vi "Read State.vi"(8 "error in (no error)":errorcluster, 11 "Monitor in":refnum<class "Monitor.lvclass">) -> (0 "error out":errorcluster, 2 "State":bool, 3 "Monitor out":refnum<class "Monitor.lvclass">)   [LabVIEW 2016, in "Monitor.lvclass"]
uses:
  Monitor.lvclass
  Monitor.lvclass/Monitor.ctl
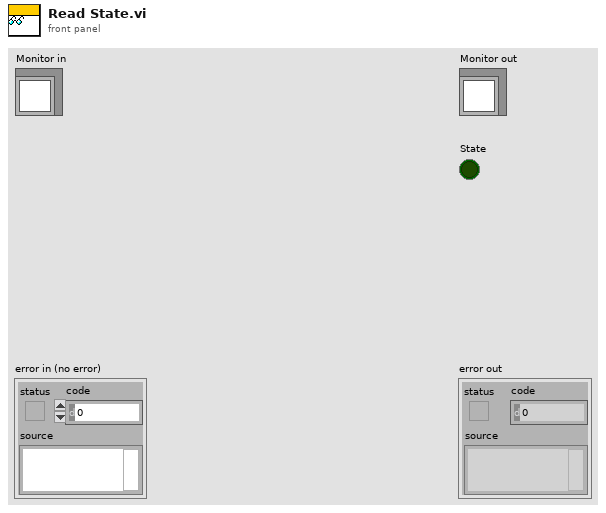
[diagram p1: front panel]
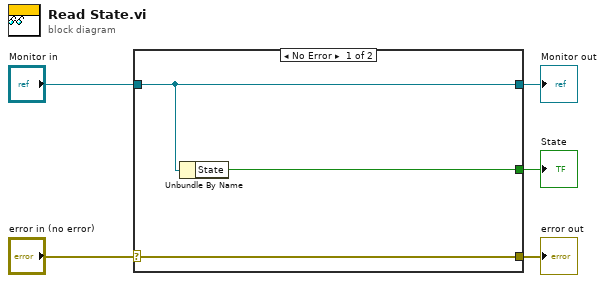
[diagram p0: block diagram]
diagram:
  n1 = case shown="No Error" "error in (no error)" {
    selector: "error in (no error)" -> [w8 w9]
    tunnel: [w8 w9] -> w4
    tunnel: [w7 w10] -> w2
    tunnel: "Monitor in" -> [w7 w10]
    tunnel: [w6 _] -> w1
    frame No Error {
      n2 = Unbundle By Name(w7) -> ("State"=w6:bool)
    }
    frame Error {
    }
  }
  "error out" <- w4
  "Monitor out" <- w2
  "State" <- w1
